vi "AddFIFO.vi"(11 "FPGA in":refnum<queue>) -> (2 "Table":string[][](array[string]), 3 "FPGA out":refnum<queue>)   [LabVIEW 2019, in "FPGA.lvlib"]
uses:
  FPGA.lvlib
  FPGA.ctl
  Commands.ctl
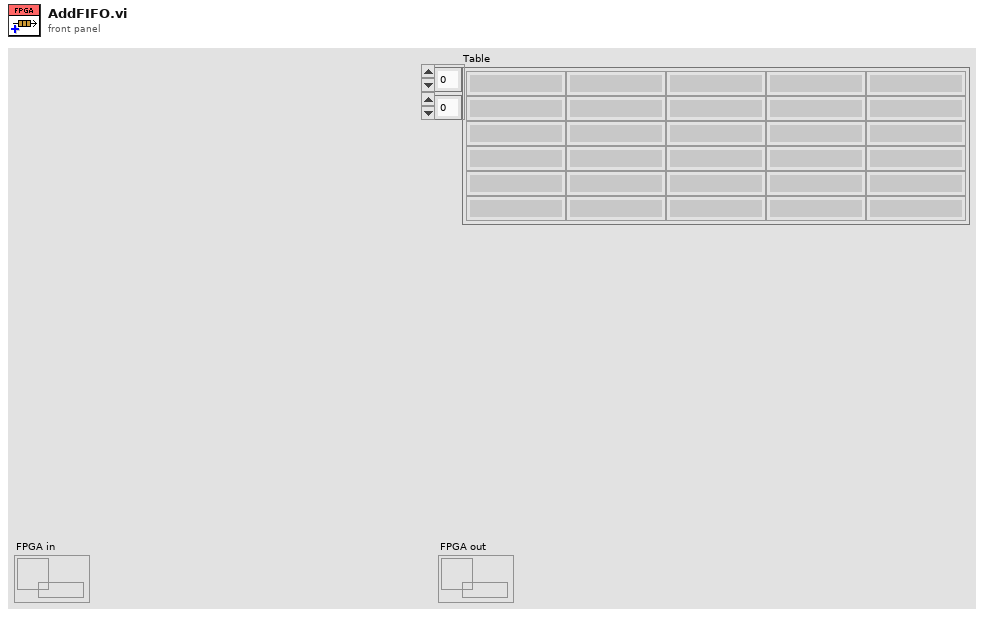
[diagram p1: front panel]
types:
  T1 = typedef "FPGA.lvlib/Commands.ctl" = string
  T2 = typedef "FPGA.lvlib/FPGA.ctl" = cluster{"Start freq. [Hz]":dbl, "Sweep duration [s]":dbl, "Freq. step [Hz]":dbl, "DAC Sample Rate":dbl, "ADC Sample Rate":dbl, "CMD port":u16, "DFAST port":u16, "CMD ID":refnum<k16>, "DFAST ID":refnum<k16>, "CMD error out":errorcluster, "FPGA IP":string, "DFAST error out ":errorcluster, "Stop freq. [Hz]":dbl, "Discrete sweep":bool, "Initial NCO":u32, "Difference NCO":i32, "step NCO":i64, "Final NCO":u32, "clocks for step":u32, "demodulation":bool, "NCO Phase Precision":u32, "NCO Sample Rate":dbl, "Time for step [s]":dbl, "NCO freq. resolution":dbl, "Sweep speed [Hz/s]":dbl, "Connected":bool, "Slew Rate [V/us]":dbl, "Parameters_ok":bool, "Amplitude [mVpp]":dbl, "Scale Factor":fxp<+,16,0>, "Acquiring":bool, "DAC-ADC Latency":u16, "Digital Gain":i32, "Number of steps":i32, "Averaging preferred":bool, "Filter Order":u32, "Settling":enum16{"99%", "99,9%"}, "FIFO":cluster{"Start freq. [Hz]":dbl, "Sweep duration [s]":dbl, "Freq. step [Hz]":dbl, "Stop freq. [Hz]":dbl, "Time for step [s]":dbl, "Amplitude [mVpp]":dbl, "Number of steps":i32}[]}
  T3 = cluster{"Start freq. [Hz]":dbl, "Sweep duration [s]":dbl, "Freq. step [Hz]":dbl, "Stop freq. [Hz]":dbl, "Time for step [s]":dbl, "Amplitude [mVpp]":dbl, "Number of steps":i32}[]
  T4 = cluster{"Start freq. [Hz]":dbl, "Sweep duration [s]":dbl, "Freq. step [Hz]":dbl, "Stop freq. [Hz]":dbl, "Time for step [s]":dbl, "Amplitude [mVpp]":dbl, "Number of steps":i32}
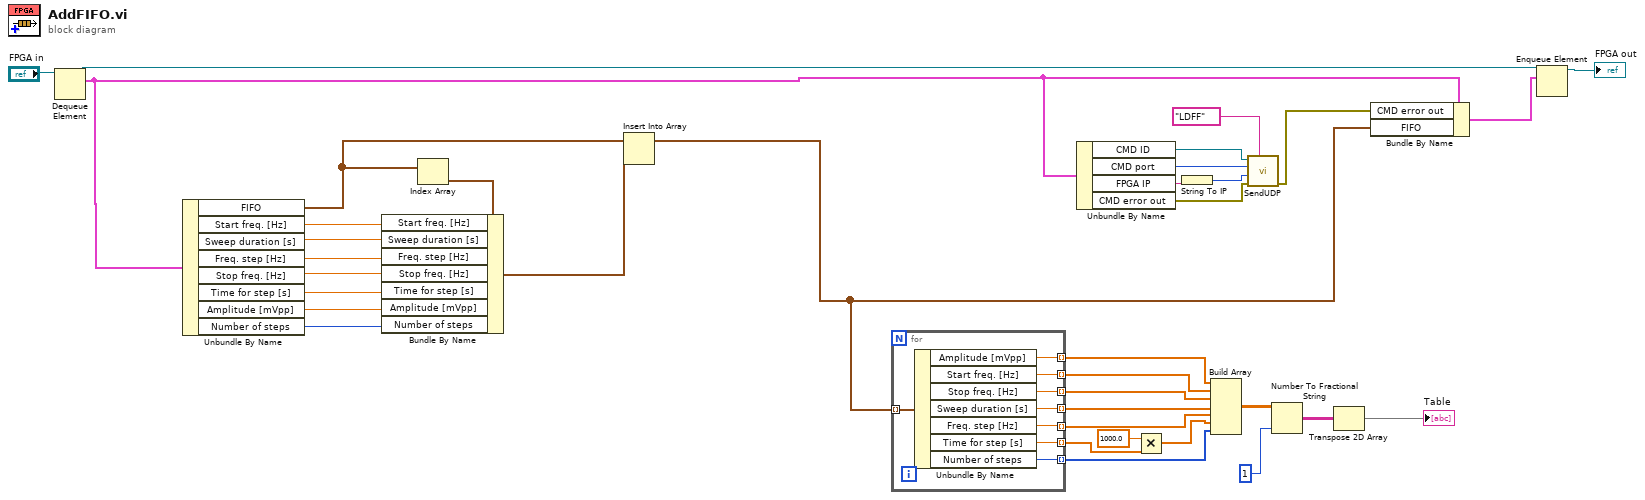
[diagram p0: block diagram]
diagram:
  n1 = Dequeue Element(queue="FPGA in") -> (queue out=w35:refnum<queue>, element=w17:T2)  [unwired: 2 in, 2 out]
  n2 = Unbundle By Name(w17) -> ("FIFO"=w33:T3, "Start freq. [Hz]"=w31:dbl, "Sweep duration [s]"=w30:dbl, "Freq. step [Hz]"=w29:dbl, "Stop freq. [Hz]"=w28:dbl, "Time for step [s]"=w27:dbl, "Amplitude [mVpp]"=w26:dbl, "Number of steps"=w25:i32)
  n3 = Index Array(array=w33) -> (element=w32:T4)  [unwired: 1 in]
  n4 = Bundle By Name(cluster=w32, "Start freq. [Hz]"=w31, "Sweep duration [s]"=w30, "Freq. step [Hz]"=w29, "Stop freq. [Hz]"=w28, "Time for step [s]"=w27, "Amplitude [mVpp]"=w26, "Number of steps"=w25) -> (w24:T4)
  n5 = Insert Into Array(array=w33, new element=w24) -> (w15:T3)  [unwired: 1 in]
  n6 = for {
    tunnel: w15 -> [w44] mode=indexing
    tunnel: [w43] -> w11 mode=indexing
    tunnel: [w42] -> w12 mode=indexing
    tunnel: [w41] -> w13 mode=indexing
    tunnel: [w40] -> w14 mode=indexing
    tunnel: [w39] -> w10 mode=indexing
    tunnel: [w38] -> w9 mode=indexing
    tunnel: [w37] -> w8 mode=indexing
    n7 = Unbundle By Name(w44) -> ("Amplitude [mVpp]"=w43:dbl, "Start freq. [Hz]"=w42:dbl, "Stop freq. [Hz]"=w41:dbl, "Sweep duration [s]"=w40:dbl, "Freq. step [Hz]"=w39:dbl, "Time for step [s]"=w38:dbl, "Number of steps"=w37:i32)
  }
  n8 = Unbundle By Name(w17) -> ("CMD ID"=w20:refnum<k16>, "CMD port"=w21:u16, "FPGA IP"=w19:string, "CMD error out"=w23:errorcluster)
  n9 = Multiply(x=1000.0, y=w9) -> (x*y=w2:dbl[])
  n10 = String To IP(1:w19) -> (0:w22:u32)
  n11 = Build Array(w11, w12, w13, w14, w10, w2, w8) -> (w7:dbl[][])
  n12 = call "SendUDP.vi"("data in"=T1 "LDFF" ("Combo Box"), "error in (no error)"=w23, "address"=w22, "port or service name"=w21, "connection ID"=w20) -> ("error out"=w16:errorcluster)  [unwired: 1 in, 5 out]
  n13 = Number To Fractional String(number=w7, precision (6)=i16 1) -> (F-format string=w5:string[][])  [unwired: 2 in]
  n14 = Transpose 2D Array(2D array=w5) -> (transposed array=→"Table":string[][])
  n15 = Bundle By Name(cluster=w17, "CMD error out"=w16, "FIFO"=w15) -> (w6:T2)
  n16 = Enqueue Element(queue=w35, element=w6) -> (queue out=→"FPGA out":refnum<queue>)  [unwired: 2 in, 2 out]
